vi "SubPanel_RFBlock_Panel_Rev11_v3.vi"(2 "error input":errorcluster, 3 "JSON file configuration?":bool, 4 "RF Block Input Array":T1[](array[typedef])) -> (0 "error output":errorcluster, 1 "RF Block Output Array":T1[](array[typedef]))   [LabVIEW 2019]
uses:
  Controls/RFBlockControl.ctl
panel:
  in  "Instrument Nickname":string="NULL"
  out "RF Block Output Echo":T1[](array[typedef])
  in  "VISA resource name":refnum<visa-resource-name>
  in  "Apply Configuration":bool
  in  "Frequency (GHz)":dbl
  in  "Power (dBm)":dbl
  in  "Power On?":bool
  in  "EXIT SUBVI":bool
  # "Instructions\nSelect Resource Under Name\nPower it on\nProvide the Frequency and Power desired\nPress \"Apply\"\nSee the output on the Echo above. If there are multiple devices configured, there will be multiple elements in the array"
  # "Nothing to see behind here"
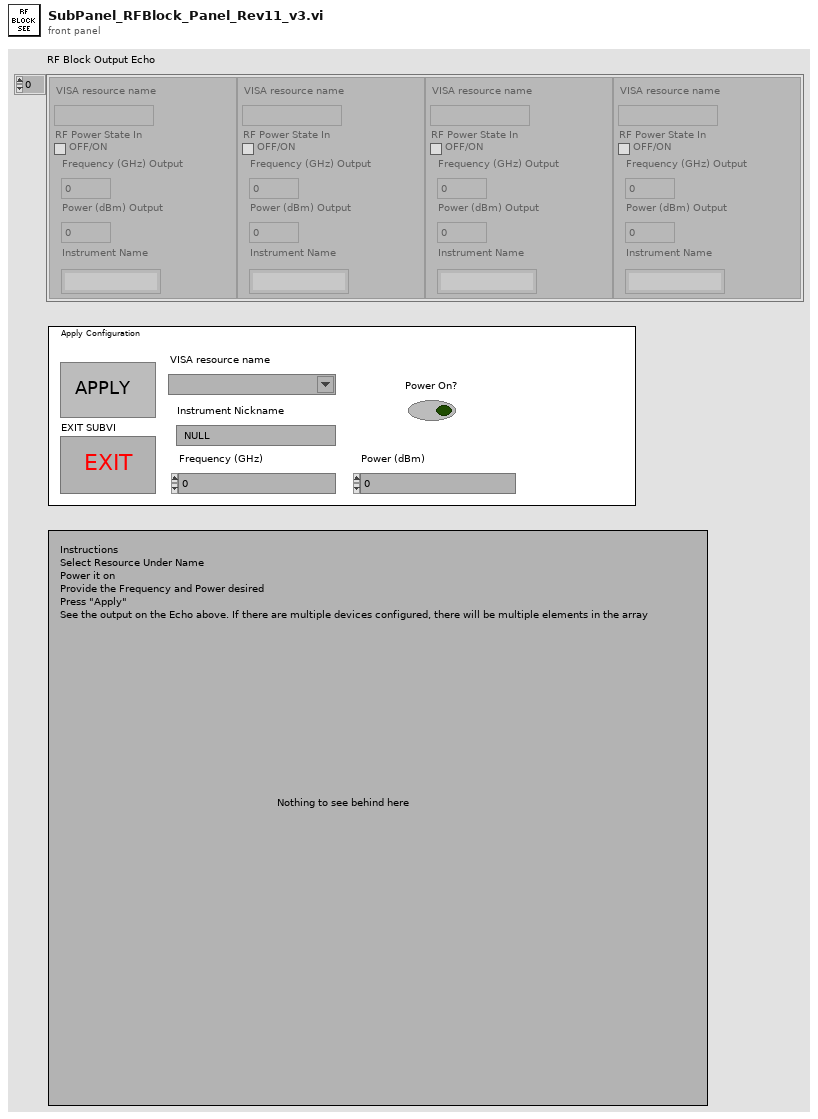
[diagram p1: front panel]
types:
  T1 = typedef "RFBlockControl.ctl" = cluster{"VISA resource name":refnum<visa-resource-name>, "RF Power State In":bool, "Frequency (GHz) Output":dbl, "Power (dBm) Output":dbl, "Instrument Name":string}
  T2 = cluster{"VISA resource name":refnum<visa-resource-name>, "Boolean out":bool, "Frequency (GHz) Output":dbl, "Power (dBm) Output":dbl, "Output Name":string}
  T3 = cluster{"VISA resource name":refnum<visa-resource-name>, "Boolean out":bool, "Frequency (GHz) Output":dbl, "Power (dBm) Output":dbl, "Instrument Name":string}
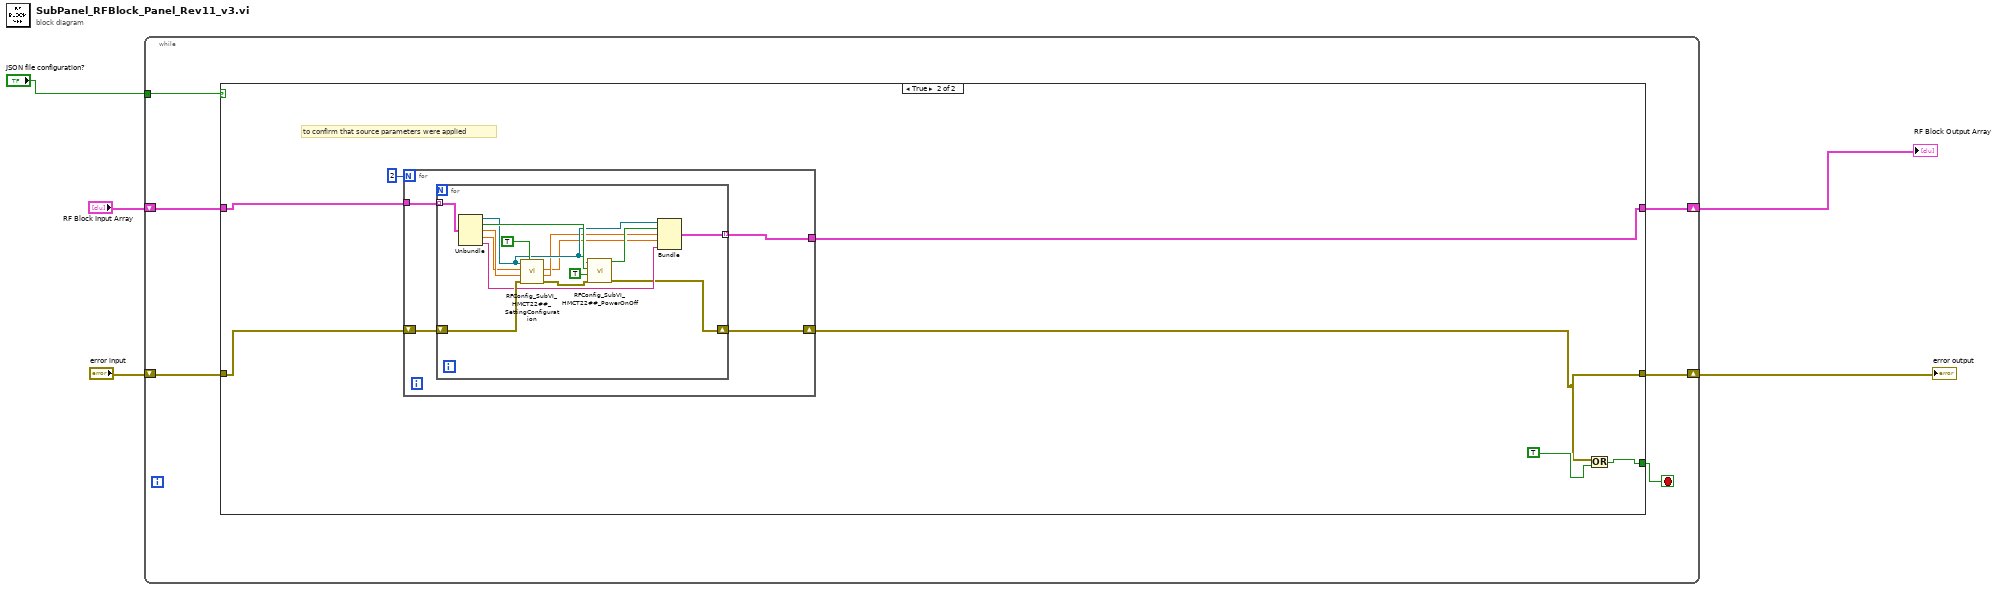
[diagram p0: block diagram]
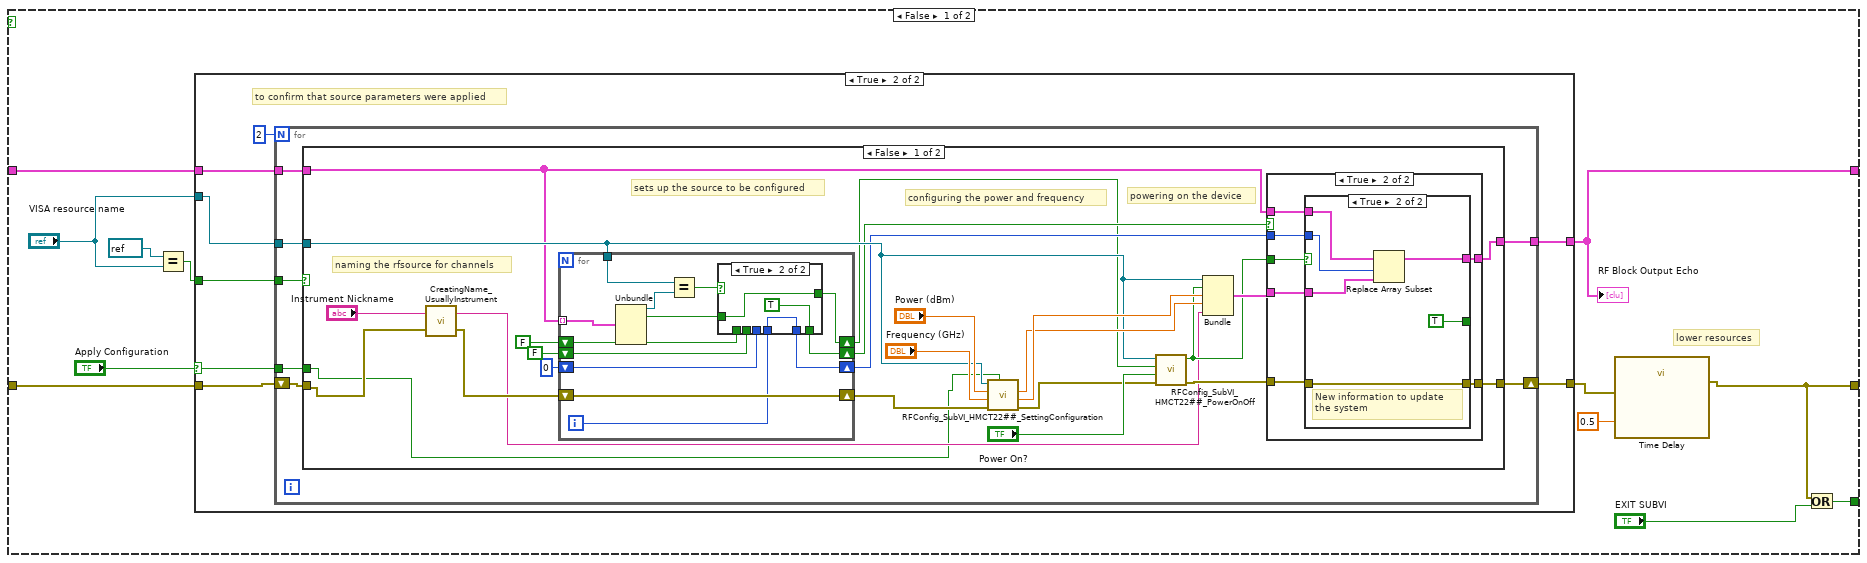
[diagram p2: hidden frame]
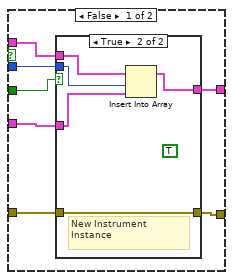
[diagram p4: hidden frame]
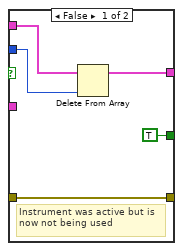
[diagram p6: hidden frame]
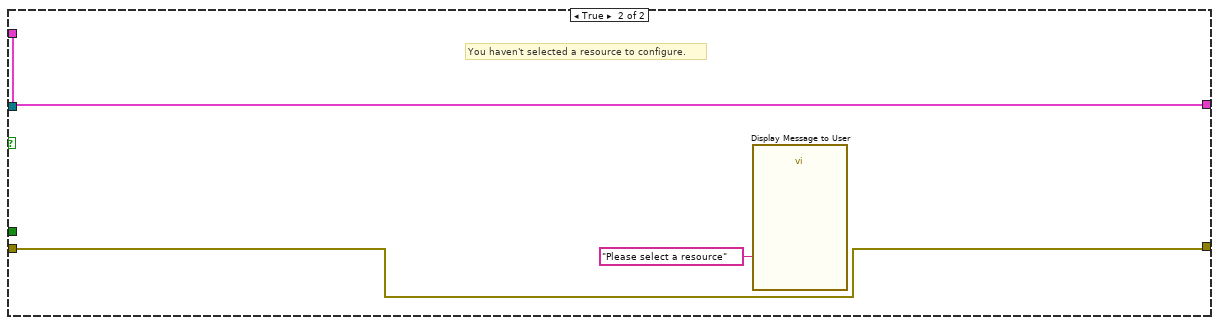
[diagram p8: hidden frame]
diagram:
  n1 = while {
    shift-right: [w8] -> w4
    shift-left: "error input" -> [w11]
    shift-right: [w9] -> w2
    shift-left: "RF Block Input Array" -> [w10]
    tunnel: "JSON file configuration?" -> [w6]
    stop <- w7 stop-if-true
    n2 = case shown="True" w6 {
      tunnel: w11 -> [w21 w123]
      tunnel: w10 -> [w16 w124]
      tunnel: [w15 w122] -> w9
      tunnel: [w14 w121] -> w8
      tunnel: [w12 w126] -> w7
      frame False {
        # "lower resources"
        n3 = Equal?(x=refnum<visa-resource-name> refnum ("VISA resource name"), y="VISA resource name") -> (x = y?=w17:bool)
        n4 = case shown="True" "Apply Configuration" {
          selector: "Apply Configuration" -> [_ w30]
          tunnel: "VISA resource name" -> [_ w33]
          tunnel: [w25 w32] -> w20
          tunnel: w21 -> [w25 w31]
          tunnel: w17 -> [_ w29]
          tunnel: w16 -> [w24 w28]
          tunnel: [w24 w27] -> w15
          frame False {
            # "Nothing happening"
          }
          frame True {
            # "to confirm that source parameters were applied"
            n5 = for {
              N: 2 -> [_]
              tunnel: w33 -> [w40]
              tunnel: w30 -> [w37]
              tunnel: w29 -> [w36]
              tunnel: w28 -> [w35]
              tunnel: [w34] -> w27
              shift-right: [w39] -> w32
              shift-left: w31 -> [w38]
              n6 = case shown="False" w36 {
                tunnel: w40 -> [w58 _]
                tunnel: [w50 w119] -> w39
                tunnel: w38 -> [w45 w119]
                tunnel: w37 -> [w41 _]
                tunnel: w35 -> [w55 w118]
                tunnel: [w48 w118] -> w34
                frame False {
                  # "naming the rfsource for channels"
                  # "powering on the device"
                  # "configuring the power and frequency"
                  # "sets up the source to be configured"
                  n7 = call "CreatingName_UsuallyInstrument.vi"("error in (no error)"=w45, "Name"="Instrument Nickname") -> ("error in (no error) 2"=w44:errorcluster, "Output Name"=w43:string)
                  n8 = for {
                    tunnel: w55 -> [w110] mode=indexing
                    shift-right: [w104] -> w59
                    shift-left: w44 -> [w104]
                    tunnel: w58 -> [w108]
                    shift-right: [w105] -> w53
                    shift-left: FALSE -> [w106]
                    shift-right: [w100] -> w52
                    shift-left: 0 -> [w101]
                    shift-right: [w98] -> w46
                    shift-left: FALSE -> [w102]
                    i -> [w99]
                    n9 = Unbundle(w110) -> ("VISA resource name"=w109:refnum<visa-resource-name>, "RF Power State In"=w103:bool)  [unwired: 3 out]
                    n10 = Equal?(x=w108, y=w109) -> (x = y?=w107:bool)
                    n11 = case shown="True" w107 {
                      tunnel: w106 -> [w113 _]
                      tunnel: [w113 TRUE] -> w105
                      tunnel: w103 -> [_ w114]
                      tunnel: w102 -> [w111 _]
                      tunnel: w101 -> [w112 _]
                      tunnel: [w112 w115] -> w100
                      tunnel: w99 -> [_ w115]
                      tunnel: [w111 w114] -> w98
                      frame False {
                      }
                      frame True {
                      }
                    }
                  }
                  n12 = call "RFConfig_SubVI_HMCT22##_SettingConfiguration.vi"("Apply Configurations"=w41, "error in (no error)"=w59, "Frequency (GHz)"="Frequency (GHz)", "Power (dBm)"="Power (dBm)", "VISA Refnum in"=w58) -> ("error out"=w62:errorcluster, "Frequency (GHz) Output"=w61:dbl, "Power (dBm) Output"=w60:dbl)  [unwired: 4 in]
                  n13 = call "RFConfig_SubVI_HMCT22##_PowerOnOff.vi"("error in (no error)"=w62, "Power On?"="Power On?", "Boolean in"=w46, "VISA Refnum in"=w58) -> ("error out"=w51:errorcluster, "Boolean out"=w49:bool)  [unwired: 6 in]
                  n14 = Bundle("VISA resource name"=w58, "Boolean out"=w49, "Frequency (GHz) Output"=w61, "Power (dBm) Output"=w60, "Output Name"=w43) -> (w54:T2)  [unwired: 1 in]
                  n15 = case shown="True" w53 {
                    tunnel: w55 -> [w71 w82]
                    tunnel: w54 -> [w70 w80]
                    tunnel: w52 -> [w69 w83]
                    tunnel: w51 -> [w66 w85]
                    tunnel: [w67 w86] -> w50
                    tunnel: w49 -> [w72 w84]
                    tunnel: [w68 w81] -> w48
                    frame False {
                      n16 = case shown="True" w72 {
                        tunnel: w71 -> [w73 w79]
                        tunnel: w70 -> [_ w78]
                        tunnel: w69 -> [_ w77]
                        tunnel: [w73 w76] -> w68
                        tunnel: [w74 w75] -> w67
                        tunnel: w66 -> [w74 w75]
                        frame False {
                          # "No instrument initialized and not powered on. Instrument not active"
                        }
                        frame True {
                          (unwired) TRUE
                          # "New Instrument Instance"
                          n17 = Insert Into Array(array=w79, index=w77, new element=w78) -> (w76:T1[])
                        }
                      }
                    }
                    frame True {
                      n18 = case shown="True" w84 {
                        tunnel: [w91 w97] -> w86
                        tunnel: w85 -> [w91 w97]
                        tunnel: w83 -> [w90 w95]
                        tunnel: w82 -> [w89 w96]
                        tunnel: [w88 w93] -> w81
                        tunnel: w80 -> [_ w94]
                        tunnel: [TRUE TRUE] -> _
                        frame False {
                          # "Instrument was active but is now not being used"
                          n19 = Delete From Array(array=w89, index=w90) -> (array with subset deleted=w88:T1[])  [unwired: 1 in, 1 out]
                        }
                        frame True {
                          # "New information to update the system"
                          n20 = Replace Array Subset(array=w96, new element=w94, index=w95) -> (w93:T1[])
                        }
                      }
                    }
                  }
                }
                frame True {
                  # "You haven't selected a resource to configure."
                  n21 = call "Display Message to User"("Message"="Please select a resource") -> ()  [unwired: 9 in, 2 out]
                }
              }
            }
          }
        }
        "RF Block Output Echo" <- w15
        n22 = call "Time Delay"("error in (no error)"=w20, "Delay Time (s)"=0.5) -> ("error out"=w14:errorcluster)  [unwired: 9 in]
        n23 = Or(x=w14, y="EXIT SUBVI") -> (x .or. y?=w12:bool)
      }
      frame True {
        # "to confirm that source parameters were applied"
        n24 = for {
          N: 2 -> [_]
          tunnel: w124 -> [w130]
          tunnel: [w128] -> w122
          shift-right: [w127] -> w121
          shift-left: w123 -> [w129]
          n25 = for {
            tunnel: w130 -> [w144] mode=indexing
            shift-right: [w132] -> w127
            shift-left: w129 -> [w140]
            tunnel: [w131] -> w128 mode=indexing
            n26 = Unbundle(w144) -> ("VISA resource name"=w137:refnum<visa-resource-name>, "RF Power State In"=w143:bool, "Frequency (GHz) Output"=w139:dbl, "Power (dBm) Output"=w138:dbl, "Instrument Name"=w133:string)
            n27 = call "RFConfig_SubVI_HMCT22##_SettingConfiguration.vi"("Apply Configurations"=TRUE, "error in (no error)"=w140, "Frequency (GHz)"=w139, "Power (dBm)"=w138, "VISA Refnum in"=w137) -> ("error out"=w141:errorcluster, "Frequency (GHz) Output"=w135:dbl, "Power (dBm) Output"=w134:dbl)  [unwired: 4 in]
            n28 = call "RFConfig_SubVI_HMCT22##_PowerOnOff.vi"("error in (no error)"=w141, "Power On?"=TRUE, "Boolean in"=w143, "VISA Refnum in"=w137) -> ("error out"=w132:errorcluster, "Boolean out"=w136:bool)  [unwired: 6 in]
            n29 = Bundle("VISA resource name"=w137, "Boolean out"=w136, "Frequency (GHz) Output"=w135, "Power (dBm) Output"=w134, "Instrument Name"=w133) -> (w131:T3)  [unwired: 1 in]
          }
        }
        n30 = Or(x=w121, y=TRUE) -> (x .or. y?=w126:bool)
      }
    }
  }
  "error output" <- w4
  "RF Block Output Array" <- w2
